vi "VI Tree.vi"   [LabVIEW 2015, in "IT6700H.lvlib"]
doc: "This is the instrument driver for the <INSTRUMENT NAME>. The VI Tree displays all the user-callable VIs of the instrument driver in an organized table."
uses:
  <instrlib>/IT6700H/IT6700H.lvlib
panel:
  # "(c) 2014 <Enter Company Name Here>.  ALL RIGHTS RESERVED."
  # "SEE DIAGRAM\nFOR VI TREE."
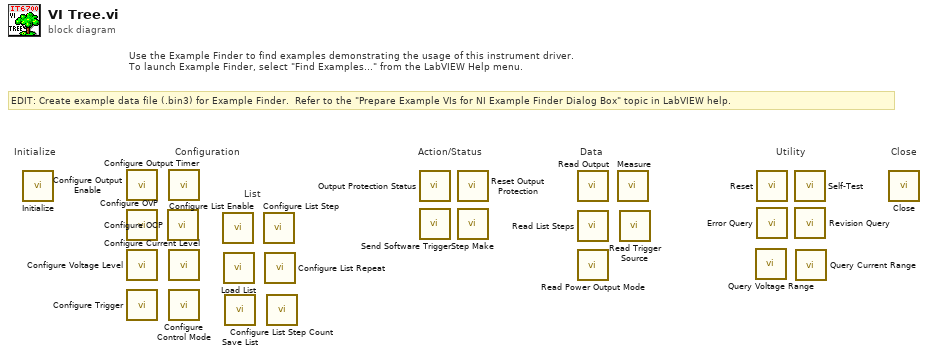
[diagram p0: block diagram]
diagram:
  # "List"
  # "EDIT: Create example data file (.bin3) for Example Finder.  Refer to the \"Prepare Example VIs for NI Example Finder Dialog Box\" topic in LabVIEW help."
  # "Use the Example Finder to find examples demonstrating the usage of this instrument driver.\nTo launch Example Finder, select \"Find Examples...\" from the LabVIEW Help menu."
  # "Configuration"
  # "Utility"
  # "Data"
  # "Action/Status"
  # "Close"
  # "Initialize"
  n1 = call <instrlib>:"Initialize.vi"() -> ()  [unwired: 10 in, 2 out]
  n2 = call <instrlib>:"Configure Output Enable.vi"() -> ()  [unwired: 9 in, 2 out]
  n3 = call <instrlib>:"Configure OVP.vi"() -> ()  [unwired: 10 in, 2 out]
  n4 = call <instrlib>:"Configure Voltage Level.vi"() -> ()  [unwired: 10 in, 2 out]
  n5 = call <instrlib>:"Configure Trigger.vi"() -> ()  [unwired: 10 in, 2 out]
  n6 = call <instrlib>:"Configure OCP.vi"() -> ()  [unwired: 10 in, 2 out]
  n7 = call <instrlib>:"Configure Output Timer.vi"() -> ()  [unwired: 10 in, 2 out]
  n8 = call <instrlib>:"Configure Current Level.vi"() -> ()  [unwired: 10 in, 2 out]
  n9 = call <instrlib>:"Configure Control Mode.vi"() -> ()  [unwired: 10 in, 2 out]
  n10 = call <instrlib>:"Configure List Enable.vi"() -> ()  [unwired: 10 in, 2 out]
  n11 = call <instrlib>:"Load List.vi"() -> ()  [unwired: 10 in, 2 out]
  n12 = call <instrlib>:"Save List.vi"() -> ()  [unwired: 10 in, 2 out]
  n13 = call <instrlib>:"Configure List Step.vi"() -> ()  [unwired: 10 in, 2 out]
  n14 = call <instrlib>:"Configure List Repeat.vi"() -> ()  [unwired: 10 in, 2 out]
  n15 = call <instrlib>:"Configure List Step Count.vi"() -> ()  [unwired: 10 in, 2 out]
  n16 = call <instrlib>:"Output Protection Status.vi"() -> ()  [unwired: 8 in, 4 out]
  n17 = call <instrlib>:"Send Software Trigger.vi"() -> ()  [unwired: 10 in, 2 out]
  n18 = call <instrlib>:"Reset Output Protection.vi"() -> ()  [unwired: 10 in, 2 out]
  n19 = call <instrlib>:"Step Make.vi"() -> ()  [unwired: 10 in, 2 out]
  n20 = call <instrlib>:"Read Output.vi"() -> ()  [unwired: 8 in, 4 out]
  n21 = call <instrlib>:"Read List Steps.vi"() -> ()  [unwired: 9 in, 3 out]
  n22 = call <instrlib>:"Read Power Output Mode.vi"() -> ()  [unwired: 9 in, 3 out]
  n23 = call <instrlib>:"Measure.vi"() -> ()  [unwired: 9 in, 3 out]
  n24 = call <instrlib>:"Read Trigger Source.vi"() -> ()  [unwired: 8 in, 3 out]
  n25 = call <instrlib>:"Query Voltage Range.vi"() -> ()  [unwired: 8 in, 4 out]
  n26 = call <instrlib>:"Reset.vi"() -> ()  [unwired: 10 in, 2 out]
  n27 = call <instrlib>:"Error Query.vi"() -> ()  [unwired: 8 in, 4 out]
  n28 = call <instrlib>:"Self-Test.vi"() -> ()  [unwired: 8 in, 4 out]
  n29 = call <instrlib>:"Revision Query.vi"() -> ()  [unwired: 8 in, 4 out]
  n30 = call <instrlib>:"Query Current Range.vi"() -> ()  [unwired: 8 in, 4 out]
  n31 = call <instrlib>:"Close.vi"() -> ()  [unwired: 11 in, 1 out]
